vi "openUDPConnection.vi"(8 "error in (no error)":errorcluster, 9 "Port:":u16=20011, 10 "SSL Vision Address:":string="127.0.0.1", 11 "Communication in":refnum<class "Communication.lvclass">) -> (0 "error out":errorcluster, 1 "connectionID out":refnum<k16>, 2 "IP Address":u32, 3 "Communication out":refnum<class "Communication.lvclass">)   [LabVIEW 2023, in "Communication.lvclass"]
uses:
  Communication.lvclass
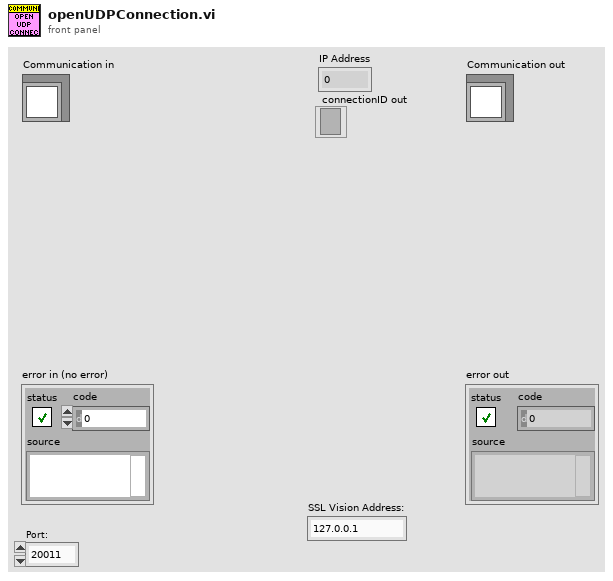
[diagram p1: front panel]
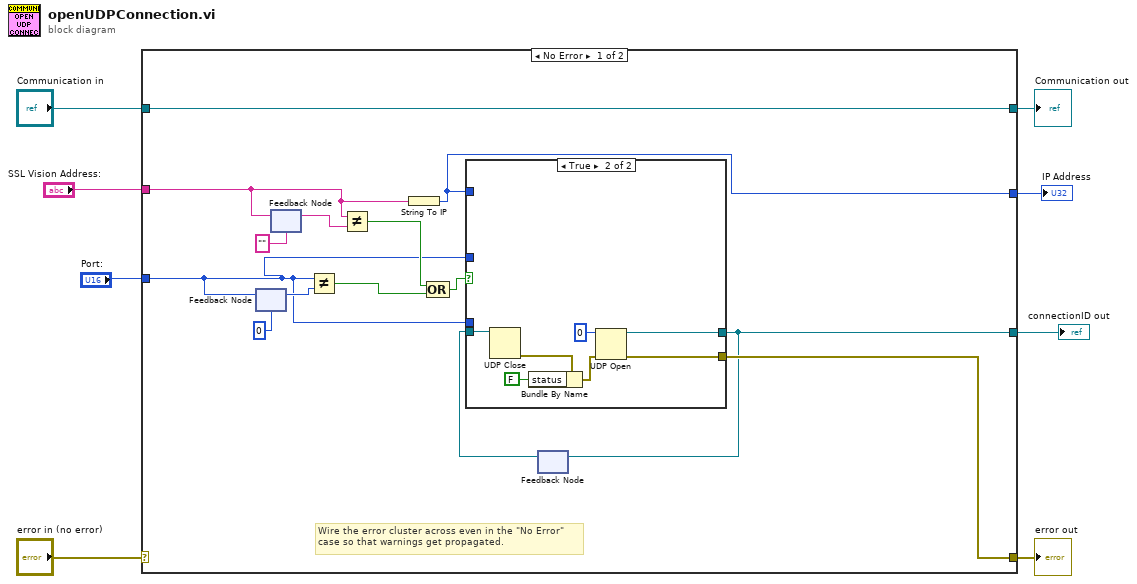
[diagram p0: block diagram]
diagram:
  n1 = case shown="No Error" "error in (no error)" {
    selector: "error in (no error)" -> [_ w32]
    tunnel: [w14 w32] -> w7
    tunnel: [w22 w31] -> w5
    tunnel: "Communication in" -> [w22 w31]
    tunnel: "SSL Vision Address:" -> [w13 _]
    tunnel: "Port:" -> [w10 _]
    tunnel: [w9 _] -> w2
    tunnel: [w12 _] -> w1
    frame No Error {
      # "Wire the error cluster across even in the \"No Error\"\ncase so that warnings get propagated."
      n2 = feedback #1(u16 0 ("Port:")) -> (w15:u16)
      n3 = feedback-in #1(w10) -> ()
      n4 = feedback #2("" ("SSL Vision Address:")) -> (w16:string)
      n5 = feedback-in #2(w13) -> ()
      n6 = Not Equal?(x=w10, y=w15) -> (x != y?=w18:bool)
      n7 = Not Equal?(x=w13, y=w16) -> (x != y?=w17:bool)
      n8 = String To IP(1:w13) -> (0:w9:u32)
      n9 = Compound Arithmetic op=OR(w17, w18) -> (w19:bool)
      n10 = feedback #3() -> (w11:refnum<k16>)  [unwired: 1 in]
      n11 = case shown="True" w19 {
        tunnel: [_ w30] -> w14
        tunnel: [w23 w25] -> w12
        tunnel: w11 -> [w23 w29]
        tunnel: w10 -> [_ _]
        tunnel: w10 -> [_ _]
        tunnel: w9 -> [_ _]
        frame False {
        }
        frame True {
          n12 = UDP Close(connection ID=w29) -> (error out=w28:errorcluster)  [unwired: 1 in, 1 out]
          n13 = Bundle By Name(cluster=w28, "status"=FALSE) -> (w27:errorcluster)
          n14 = UDP Open(8:w27, 11:u16 0 ("port")) -> (port=w25:refnum<k16>, 0:w30:errorcluster)  [unwired: 3 in, 1 out]
        }
      }
      n15 = feedback-in #3(w12) -> ()
    }
    frame Error {
    }
  }
  "error out" <- w7
  "Communication out" <- w5
  "IP Address" <- w2
  "connectionID out" <- w1
